vi "MDPtr Pack Waveform.vi"(7 "Copies Count(1)":i32=1, 9 "String Attribute":string, 10 "error in (no error)":errorcluster, 11 "waveform":waveform(dbl)) -> (2 "error out":errorcluster, 3 "HexStrPtr":T1)   [LabVIEW 2017, in "MDPtr.lvlib"]
uses:
  MDPtr.lvlib
  MDPtr TypeDef/MDPtr.ctl
  MDPtr TypeDef/MDPtr DataFrame-Waveform.ctl
  MDPtr TypeDef/MDPtr DataFrame-Common.ctl
  MDPtr TypeDef/MDPtr SupportedDataTypeDef.ctl
  _MDPtrMgr/MDPtrMgr.lvclass
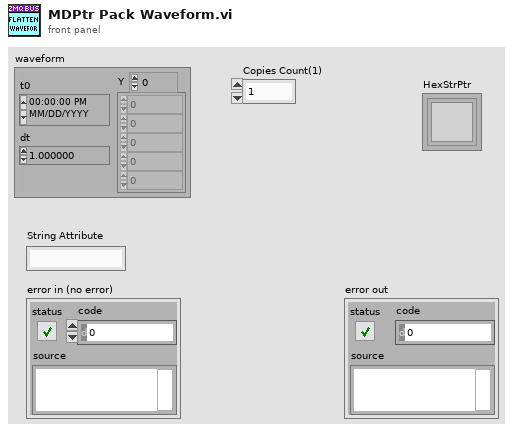
[diagram p1: front panel]
types:
  T1 = typedef "MDPtr.lvlib/MDPtr.ctl" = refnum<k1>
  T2 = typedef "MDPtr.lvlib/MDPtr DataFrame-Waveform.ctl" = cluster{"Common":T3, "DVR":refnum<data-value>}
  T3 = typedef "MDPtr.lvlib/MDPtr DataFrame-Common.ctl" = cluster{"Data Type":T4, "Copy Count":i32, "String Attribute":string}
  T4 = typedef "MDPtr.lvlib/MDPtr SupportedDataTypeDef.ctl" = enum16{"<Invalid>", "<User 0>", "<User 1>", "<User 2>", "<User 3>", "<User 4>", "Memory", "Waveform", "Waveform Arr", "Double Arr", "String Arr"}
  T5 = typedef "MDPtr.lvlib/Def-MDPtrQueue.ctl" = refnum<queue>
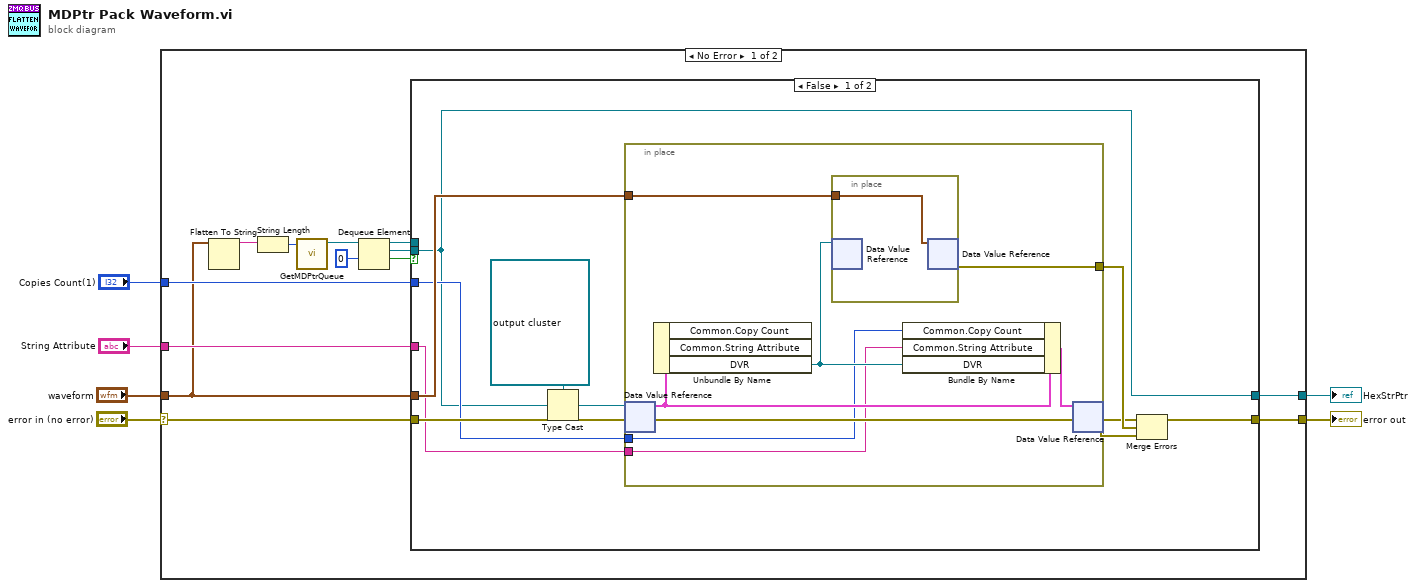
[diagram p0: block diagram]
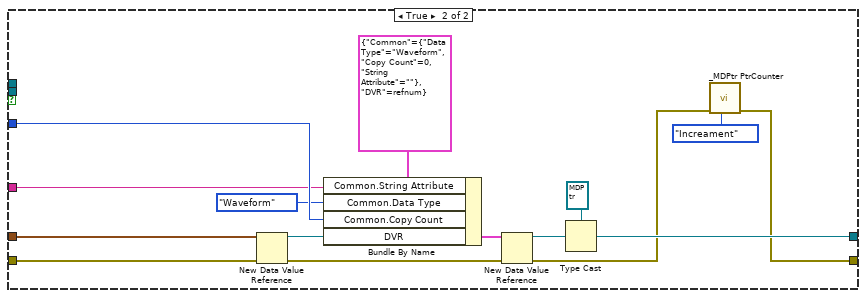
[diagram p2: hidden frame]
diagram:
  n1 = case shown="No Error" "error in (no error)" {
    selector: "error in (no error)" -> [w19 w53]
    tunnel: [w11 w53] -> w1
    tunnel: "waveform" -> [w9 _]
    tunnel: [w18 _] -> w4
    tunnel: "Copies Count(1)" -> [w17 _]
    tunnel: "String Attribute" -> [w16 _]
    frame No Error {
      n2 = Flatten To String(anything=w9) -> (data string=w8:string)  [unwired: 3 in, 2 out]
      n3 = String Length(string=w8) -> (length=w7:i32)
      n4 = call "GetMDPtrQueue.vi"("MemoryLength"=w7) -> ("MDPtrQueue"=w10:T5)  [unwired: 9 in, 1 out]
      n5 = Dequeue Element(queue=w10, timeout in ms (-1)=0) -> (queue out=w13:T5, element=w12:T1, timed out?=w14:bool)  [unwired: 1 in, 1 out]
      n6 = case shown="False" w14 {
        tunnel: w19 -> [w25 w51]
        tunnel: [w24 w38] -> w11
        tunnel: [w20 w48] -> w18
        tunnel: w17 -> [w21 w46]
        tunnel: w16 -> [w22 w42]
        tunnel: w9 -> [w23 w41]
        tunnel: w13 -> [_ _]
        tunnel: w12 -> [w20 _]
        frame False {
          n7 = Type Cast(type=refnum<data-value> refnum ("data value reference"), x=w20) -> (*(type *) &x=w29:refnum<data-value>)
          n8 = in-place {
            in-place-border: [w33] -> w27
            in-place-border: w23 -> [w32]
            in-place-border: w22 -> [w31]
            in-place-border: w21 -> [w30]
            n9 = in-place-dvr #1(w29) -> (w36:T2)  [unwired: 1 out]
            n10 = Unbundle By Name(w36) -> ("DVR"=w34:refnum<data-value>)  [unwired: 2 out]
            n11 = in-place {
              in-place-border: w32 -> [w37]
              n12 = in-place-dvr #2(w34) -> ()  [unwired: 2 out]
              n13 = in-place-dvr #2(w37) -> (w33:errorcluster)  [unwired: 1 out]
            }
            n14 = Bundle By Name(cluster=w36, "Common.Copy Count"=w30, "Common.String Attribute"=w31, "DVR"=w34) -> (w35:T2)
            n15 = in-place-dvr #1(w35) -> (w26:errorcluster)  [unwired: 1 out]
          }
          n16 = Merge Errors(w25, w27, w26) -> (w24:errorcluster)
        }
        frame True {
          n17 = New Data Value Reference(data value=w41, error in=w51) -> (data value reference=w47:refnum<data-value>, error out=w50:errorcluster)
          n18 = Bundle By Name(cluster=T2 {"Common"={"Data Type"=enum."Waveform", "Copy Count"=0, "String Attribute"=""}, "DVR"=refnum} ("DataFrame-Waveform"), "Common.String Attribute"=w42, "Common.Data Type"=MDPtr_SupportedDataTypeDef."Waveform" ("Data Type"), "Common.Copy Count"=w46, "DVR"=w47) -> (w52:T2)
          n19 = New Data Value Reference(data value=w52, error in=w50) -> (data value reference=w49:refnum<data-value>, error out=w39:errorcluster)
          n20 = Type Cast(type=T1 refnum ("MDPtr"), x=w49) -> (*(type *) &x=w48:T1)
          n21 = call "_MDPtr PtrCounter.vi"("Oper(Get)"=enum16{"GET", "Increament", "decreament"}."Increament", "error in (no error)"=w39) -> ("error out"=w38:errorcluster)  [unwired: 8 in, 1 out]
        }
      }
    }
    frame Error {
    }
  }
  "HexStrPtr" <- w4
  "error out" <- w1
